vi "setIcon.vi"(8 "Error In":errorcluster, 10 "icon":refnum<class "QIcon.lvclass">, 11 "QAbstractButton In":refnum<class "QAbstractButton.lvclass">) -> (0 "Error Out":errorcluster, 3 "QAbstractButton Out":refnum<class "QAbstractButton.lvclass">)   [LabVIEW 2014, in "QAbstractButton.lvclass"]
doc: "LabVIEW-specific documentation is not yet available. See <b>http://doc.qt.io/qt-5/QAbstractButton.html#setIcon</b>"
uses:
  QAbstractButton.lvclass
  Qt GUI/QIcon/QIcon.lvclass
  LQ Core/LQIdentity/LQIdentity.lvclass/LQIdentity.ctl
  LQ Core/LQSerialData/LQSerialData.lvclass/LQSerialData.ctl
  LQ Core/LQ Core.lvlib
  LQ Core/LQIdentity/LQIdentity.lvclass
  LQ Core/LQSerialData/LQSerialData.lvclass
panel:
  # "Copyright (c) 2016 Sze Howe Koh\n\nThis Source Code Form is subject to the terms of the Mozilla Public\nLicense, v. 2.0. If a copy of the MPL was not distributed with this\nfile, You can obtain one at http://mozilla.org/MPL/2.0/."
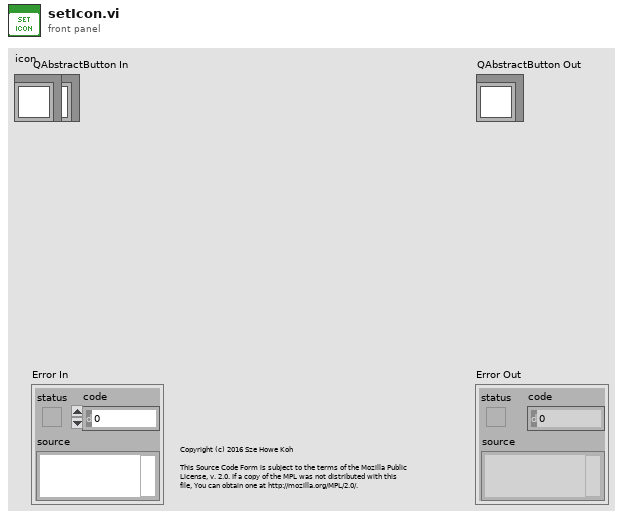
[diagram p1: front panel]
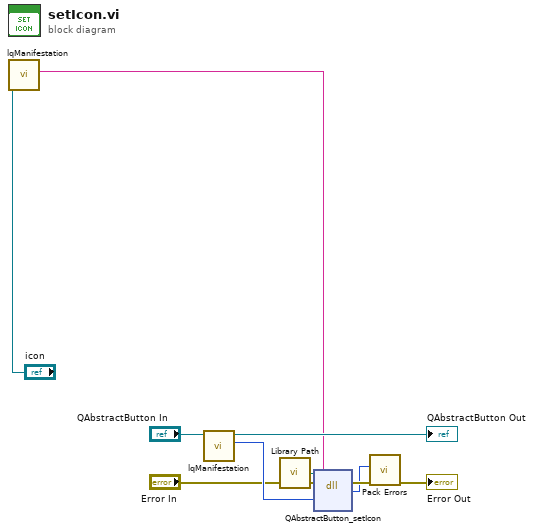
[diagram p0: block diagram]
diagram:
  n1 = call "lqManifestation.vi"("LQSerialData in"="icon") -> ("Manifestation"=w1:string)  [unwired: 9 in, 1 out]
  n2 = call "lqManifestation.vi"("LQIdentity in"="QAbstractButton In") -> ("Manifestation"=w7:u64, "LQIdentity out"=→"QAbstractButton Out":refnum<class "QAbstractButton.lvclass">)  [unwired: 9 in]
  n3 = call "Library Path.vi"() -> ("Library Path"=w8:path)
  n4 = dll-call lib="?" fn="QAbstractButton_setIcon"(path in=w8, error in="Error In", "_instance"=w7, "icon"=w1) -> (error out=w5:errorcluster, w3:i32)  [unwired: 3 in, 1 out]
  n5 = call "Pack Errors.vi"("Error In"=w5, "Error Code"=w3) -> ("Error Out"=→"Error Out":errorcluster)  [unwired: 9 in]
